vi "Initialize System.vi"(8 "error in (no error)":errorcluster, 10 "Subsystem I/O Attributes":T3[](array[typedef]), 11 "System Configuration In":T1) -> (0 "error out":errorcluster, 3 "System Configuration Out":T1)   [LabVIEW 2024]
doc: "Initializes the server, creates the server process in the shared variable engine, and applies server configurations."
uses:
  Controls/Server/System Configuration.ctl
  Controls/Server/Subsystem Configuration.ctl
  Controls/Server/Subsystem IO Attributes.ctl
  Controls/Server/Subsystem IO Logging Attributes.ctl
  Controls/Server/Subsystem IO Alarm Attributes.ctl
  <vilib>/lvdsc/NI_DSC.lvlib
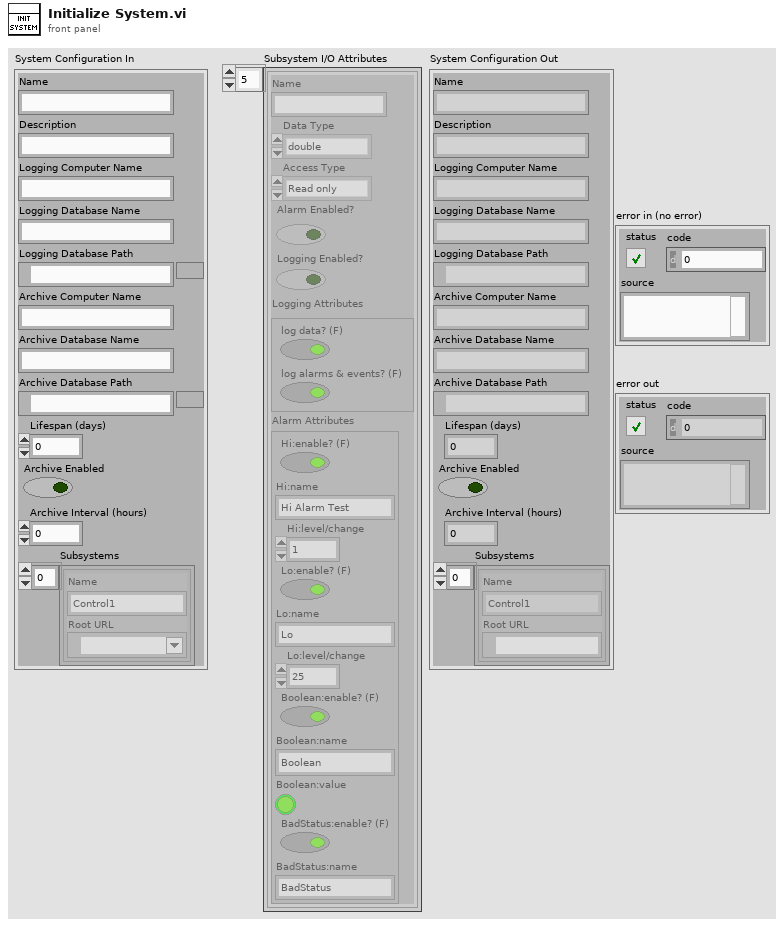
[diagram p1: front panel]
types:
  T1 = typedef "System Configuration.ctl" = cluster{"Name":string, "Description":string, "Logging Computer Name":string, "Logging Database Name":string, "Logging Database Path":path, "Archive Computer Name":string, "Archive Database Name":string, "Archive Database Path":path, "Lifespan (days)":u32, "Archive Enabled":bool, "Archive Interval (hours)":u32, "Subsystems":T2[]}
  T2 = typedef "Subsystem Configuration.ctl" = cluster{"Name":string, "Root URL":refnum<k21>}
  T3 = typedef "Subsystem IO Attributes.ctl" = cluster{"Name":string, "Data Type":enum32{"u32BitField", "bool", "double", "string", "int8", "uint8", "int16", "uint16", "int32", "uint32", "int64", "uint64", "single", "double waveform", "int16 waveform", "array of boolean", "array of int8", "array of uint8", "array of int16", "array of uint16", "array of int32", "array of uint32", "array of int64", "array of uint64", "array of single", "array of double", "array of double waveform", "array of int16 waveform", "array of string", "variant", "timestamp", "fixed point", "custom"}, "Access Type":enum32{"Read only", "Write only", "Read/write"}, "Alarm Enabled?":bool, "Logging Enabled?":bool, "Logging Attributes":T4, "Alarm Attributes":T5}
  T4 = typedef "Subsystem IO Logging Attributes.ctl" = cluster{"log data? (F)":bool, "log alarms & events? (F)":bool}
  T5 = typedef "Subsystem IO Alarm Attributes.ctl" = cluster{"Hi:enable? (F)":bool, "Hi:name":string, "Hi:level/change":dbl, "Lo:enable? (F)":bool, "Lo:name":string, "Lo:level/change":dbl, "Boolean:enable? (F)":bool, "Boolean:name":string, "Boolean:value":bool, "BadStatus:enable? (F)":bool, "BadStatus:name":string}
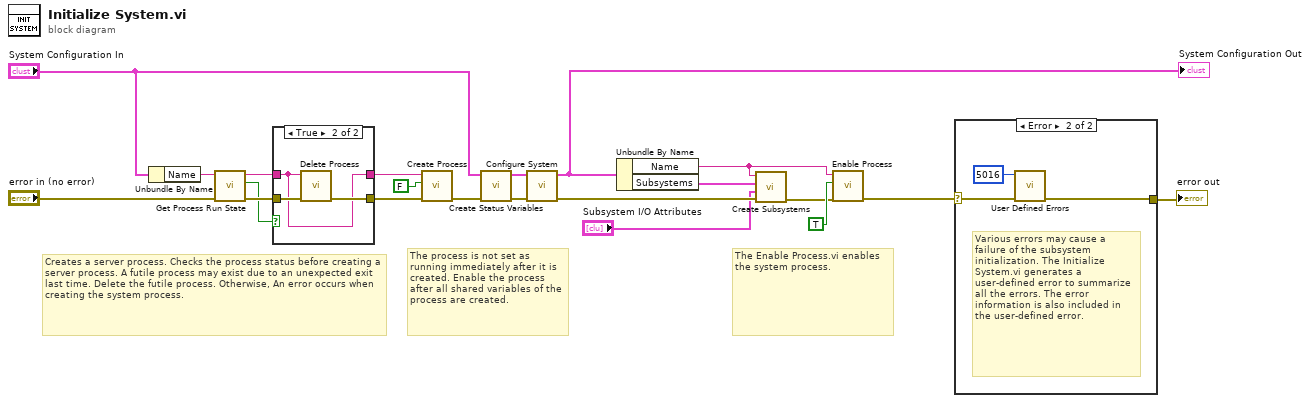
[diagram p0: block diagram]
diagram:
  # "The Enable Process.vi enables the system process."
  # "The process is not set as running immediately after it is created. Enable the process after all shared variables of the process are created."
  # "Creates a server process. Checks the process status before creating a server process. A futile process may exist due to an unexpected exit last time. Delete the futile process. Otherwise, An error occurs when creating the system process."
  n1 = Unbundle By Name("System Configuration In") -> ("Name"=w19:string)
  n2 = call <vilib>:"Get Process Run State.vi"("error in (no error)"="error in (no error)", "process name"=w19) -> ("error out"=w17:errorcluster, "exists?"=w10:bool, "process name out"=w16:string)  [unwired: 6 in, 1 out]
  n3 = case shown="True" w10 {
    tunnel: w17 -> [w23 w26]
    tunnel: w16 -> [w22 w24]
    tunnel: [w23 w25] -> w15
    tunnel: [w22 w24] -> w9
    frame False {
    }
    frame True {
      n4 = call <vilib>:"Delete Process.vi"("error in (no error)"=w26, "process name"=w24) -> ("error out"=w25:errorcluster)  [unwired: 9 out]
    }
  }
  n5 = call <vilib>:"Create Process.vi"("error in (no error)"=w15, "run?"=FALSE, "process name"=w9) -> ("error out"=w14:errorcluster)  [unwired: 3 in, 5 out]
  n6 = call "Create Status Variables.vi"("error in (no error)"=w14, "System Configuration"="System Configuration In") -> ("error out"=w13:errorcluster, "dup System Configuration"=w8:T1)  [unwired: 8 in]
  n7 = call "Configure System.vi"("error in (no error)"=w13, "System Configuration"=w8) -> ("error out"=w5:errorcluster, "dup System Configuration"=w1:T1)  [unwired: 8 in]
  "System Configuration Out" <- w1
  n8 = Unbundle By Name(w1) -> ("Name"=w2:string, "Subsystems"=w6:T2[])
  n9 = call "Create Subsystems.vi"("error in (no error)"=w5, "Subsystem I/O Attributes"="Subsystem I/O Attributes", "Subsystems"=w6, "System Name"=w2) -> ("error out"=w3:errorcluster)  [unwired: 7 in]
  n10 = call <vilib>:"Enable Process.vi"("error in (no error)"=w3, "run?"=TRUE, "process name"=w2) -> ("error out"=w12:errorcluster)  [unwired: 7 in, 1 out]
  n11 = case shown="Error" w12 {
    selector: w12 -> [w27 w29]
    tunnel: [w27 w28] -> w11
    frame No Error {
    }
    frame Error {
      # "Various errors may cause a failure of the subsystem initialization. The Initialize System.vi generates a user-defined error to summarize all the errors. The error information is also included in the user-defined error."
      n12 = call "User Defined Errors.vi"("error in (no error)"=w29, "Error Code (0)"=5016 ("error code (0)")) -> ("error out"=w28:errorcluster)  [unwired: 9 in]
    }
  }
  "error out" <- w11
